vi "_16_Sample_qsns_05[14].vi"() -> ()   [LabVIEW 2020]
panel:
  out "Numeric":i32
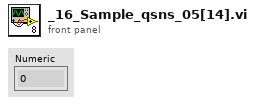
[diagram p1: front panel]
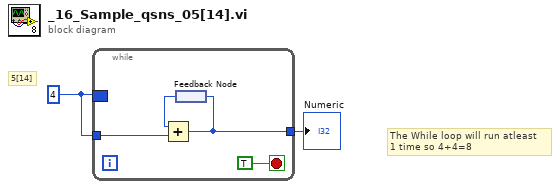
[diagram p0: block diagram]
diagram:
  w2 = 4
  # "5[14]"
  # "The While loop will run atleast \n1 time so 4+4=8"
  n1 = while {
    border: w2 -> [_]
    tunnel: w2 -> [w6]
    tunnel: [w4] -> w1
    stop <- TRUE stop-if-true
    n2 = feedback #1() -> (w5:i32)
    n3 = Add(x=w5, y=w6) -> (x+y=w4:i32)
    n4 = feedback-in #1(w4) -> ()
  }
  "Numeric" <- w1
